vi "wait_with_status.vi"(4 "stat ref":refnum<vi>, 6 "stop ref":refnum<vi>, 8 "error in":errorcluster, 9 "comment":string, 10 "skip ref":refnum<vi>, 11 "ms to wait":i32) -> (0 "error out":errorcluster)   [LabVIEW 2013]
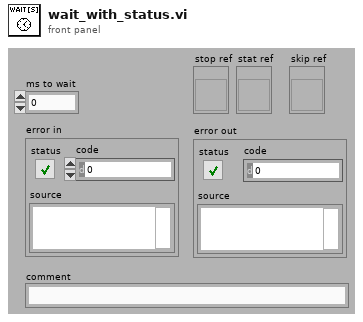
[diagram p1: front panel]
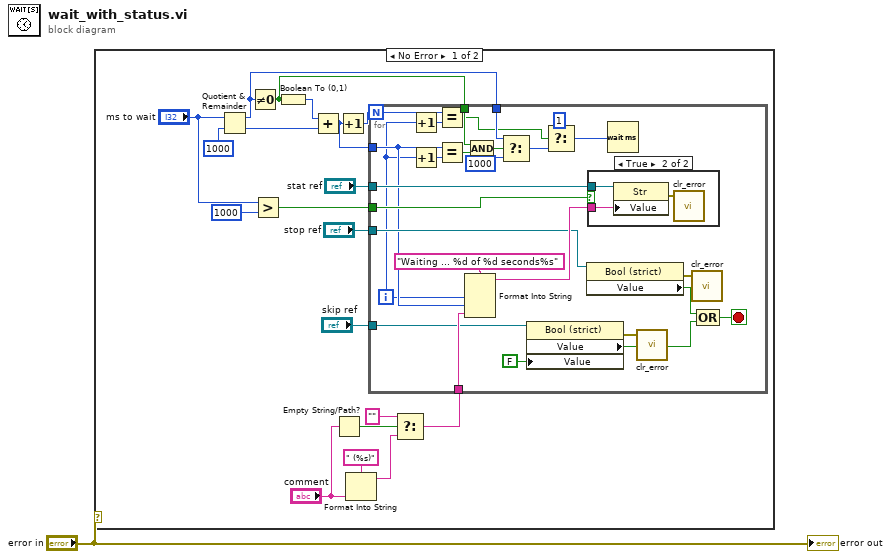
[diagram p0: block diagram]
diagram:
  n1 = case shown="No Error" "error in" {
    frame No Error {
      n2 = Quotient & Remainder(x="ms to wait", y=1000) -> (x-y*floor(x/y)=w10:i32, floor(x/y)=w11:i32)
      n3 = Not Equal To 0?(x=w10) -> (x != 0?=w9:bool)
      n4 = Greater?(x="ms to wait", y=1000) -> (0:w5:bool)
      n5 = Boolean To (0,1)(Boolean=w9) -> (0, 1=w8:i16)
      n6 = Add(x=w8, y=w11) -> (x+y=w3:i32)
      n7 = Empty String/Path?(string/path="comment") -> (empty?=w17:bool)
      n8 = Increment(x=w3) -> (x+1=w4:i32)
      n9 = Format Into String(format string=" (%s)", "comment") -> (resulting string=w14:string)  [unwired: 2 in, 1 out]
      n10 = Select(t="", s=w17, f=w14) -> (s? t:f=w16:string)
      n11 = for {
        N: w4 -> [w33]
        tunnel: "stat ref" -> [w47]
        tunnel: "stop ref" -> [w44]
        tunnel: w16 -> [w42]
        tunnel: w10 -> [w40]
        tunnel: w9 -> [w37]
        tunnel: w5 -> [w35]
        tunnel: w3 -> [w34]
        tunnel: "skip ref" -> [w26]
        i -> [w31]
        stop <- w22 stop-if-true
        n12 = Increment(x=w31) -> (x+1=w32:i32)
        n13 = Increment(x=w31) -> (x+1=w39:i32)
        n14 = Equal?(x=w33, y=w32) -> (x = y?=w29:bool)
        n15 = Equal?(x=w34, y=w39) -> (x = y?=w38:bool)
        n16 = Format Into String(format string="Waiting ... %d of %d seconds%s", w31, w34, w42) -> (resulting string=w46:string)  [unwired: 2 in, 1 out]
        n17 = And(x=w37, y=w38) -> (x .and. y?=w36:bool)
        n18 = Select(t=w40, s=w36, f=u32 1000 ("milliseconds to wait")) -> (s? t:f=w30:u32)
        n19 = property class="Bool (strict)"(reference=w26, "Value"=FALSE) -> (error out=w25:errorcluster, "Value"=w23:bool)  [unwired: 1 in, 1 out]
        n20 = Select(t=u32 1, s=w29, f=w30) -> (s? t:f=w27:u32)
        n21 = property class="Bool (strict)"(reference=w44) -> (error out=w43:errorcluster, "Value"=w24:bool)  [unwired: 1 in, 1 out]
        n22 = case shown="True" w35 {
          tunnel: w47 -> [_ w50]
          tunnel: w46 -> [_ w49]
          frame False {
          }
          frame True {
            n23 = property class="Str"(reference=w50, "Value"=w49) -> (error out=w48:errorcluster)  [unwired: 1 in, 1 out]
            n24 = call "clr_error.vi"("error in (no error)"=w48) -> ()  [unwired: 4 in, 1 out]
          }
        }
        n25 = Wait (ms)(milliseconds to wait=w27) -> ()  [unwired: 1 out]
        n26 = call "clr_error.vi"("error in (no error)"=w25) -> ()  [unwired: 4 in, 1 out]
        n27 = call "clr_error.vi"("error in (no error)"=w43) -> ()  [unwired: 4 in, 1 out]
        n28 = Compound Arithmetic op=OR(w24, w23) -> (w22:bool)
      }
    }
    frame Error {
    }
  }
  "error out" <- "error in"
